vi "parse simple scan cluster.vi"(9 "variable":string, 10 "device":string, 11 "Scan setup":T1={"Scan Start"=1.0, "Scan End"=10.0, "Scan Step Size"=1.0, "# Shots Each Step"=10, "single direction?"=TRUE} {"Scan Start" format="%#.9p"; "Scan End" format="%#.9p"; "Scan Step Size" format="%#.9p"}) -> (1 "# shots":i32, 2 "bin group":i32[](array[numeric]), 3 "State(s) out":string)   [LabVIEW 2020]
uses:
  scan parameters.ctl
  <userlib>/_OpenG.lib/array/array.llb/Remove Duplicates from 1D Array (DBL)__ogtk.vi
panel:
  out "# shots 2":dbl
  out "vals to scan":dbl[](array[numeric])
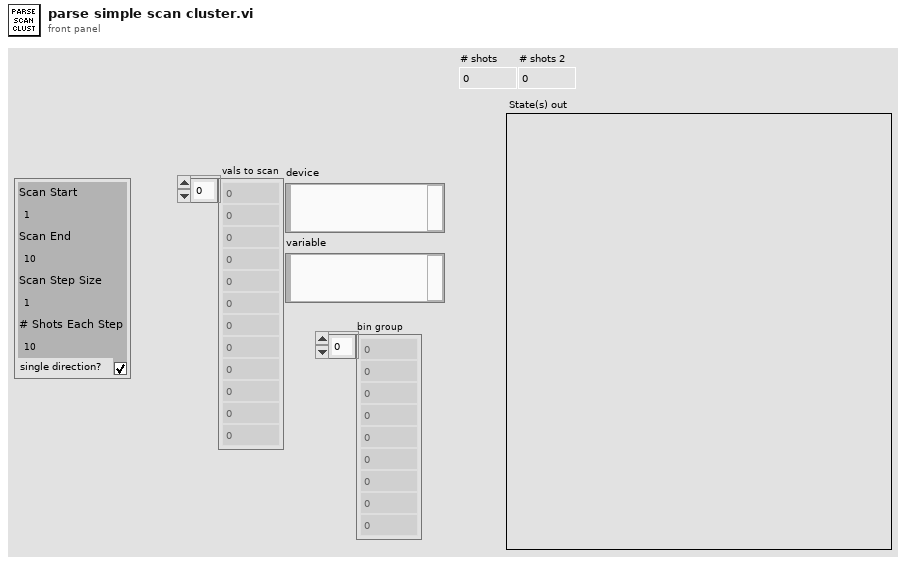
[diagram p1: front panel]
types:
  T1 = typedef "scan parameters.ctl" = cluster{"Scan Start":dbl, "Scan End":dbl, "Scan Step Size":dbl, "# Shots Each Step":u32, "single direction?":bool}
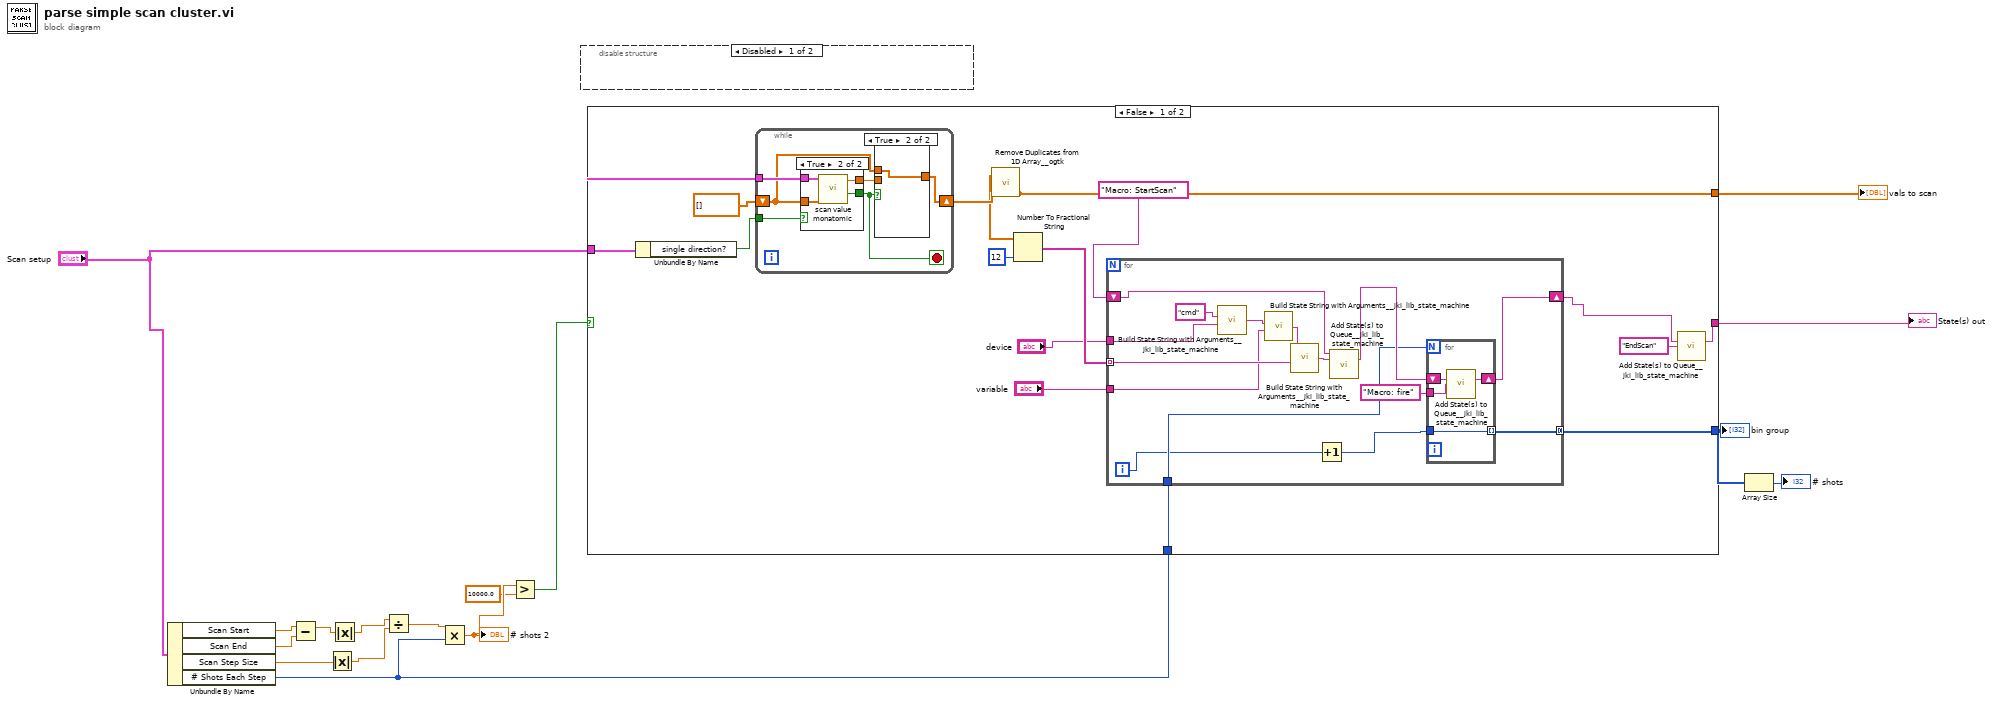
[diagram p0: block diagram]
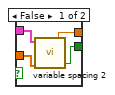
[diagram p2: hidden frame]
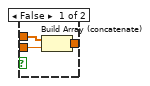
[diagram p3: hidden frame]
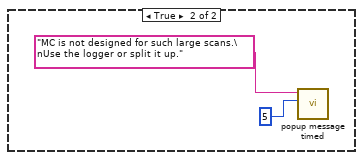
[diagram p4: hidden frame]
diagram:
  n1 = Unbundle By Name("Scan setup") -> ("Scan Start"=w12:dbl, "Scan End"=w11:dbl, "Scan Step Size"=w10:dbl, "# Shots Each Step"=w5:u32)
  n2 = Subtract(x=w12, y=w11) -> (x-y=w9:dbl)
  n3 = Absolute Value(x=w10) -> (abs(x)=w7:dbl)
  n4 = Absolute Value(x=w9) -> (abs(x)=w8:dbl)
  n5 = Divide(x=w8, y=w7) -> (x/y=w6:dbl)
  n6 = Multiply(x=w6, y=w5) -> (x*y=w4:dbl)
  "# shots 2" <- w4
  n7 = Greater?(x=w4, y=10000.0) -> (0:w2:bool)
  n8 = disable-structure shown="Disabled" {
    frame Disabled {
    }
    frame Enabled {
    }
  }
  n9 = case shown="False" w2 {
    tunnel: "Scan setup" -> [w31 _]
    tunnel: [w30 _] -> w15
    tunnel: [w24 _] -> w14
    tunnel: w5 -> [w20 _]
    tunnel: [w17 _] -> w1
    frame False {
      n10 = Unbundle By Name(w31) -> ("single direction?"=w25:bool)
      n11 = while {
        tunnel: w31 -> [w37]
        shift-right: [w34] -> w30
        shift-left: dbl[] [] ("parameter vals scanned") -> [w36]
        tunnel: w25 -> [w32]
        stop <- w33 stop-if-true
        n12 = case shown="True" w32 {
          tunnel: w37 -> [w41 w45]
          tunnel: w36 -> [w40 w44]
          tunnel: [w39 w43] -> w35
          tunnel: [w38 w42] -> w33
          frame False {
            n13 = call "variable spacing 2.vi"("shot times"=w40, "Scan parameters"=w41) -> ("quit"=w38:bool, "time aimed"=w39:dbl)  [unwired: 2 in, 1 out]
          }
          frame True {
            n14 = call "scan value monatomic.vi"("parameter vals scanned"=w44, "Scan parameters"=w45) -> ("scan complete"=w42:bool, "Next Value"=w43:dbl)  [unwired: 7 in, 1 out]
          }
        }
        n15 = case shown="True" w33 {
          tunnel: w36 -> [w48 w49]
          tunnel: w35 -> [w47 _]
          tunnel: [w46 w49] -> w34
          frame False {
            n16 = Build Array (concatenate)(w48, w47) -> (w46:dbl[])
          }
          frame True {
          }
        }
      }
      n17 = call-poly <userlib>:"Remove Duplicates from 1D Array__ogtk.vi"("Input Array"=w30) -> ("Output Array"=w29:dbl[])  [unwired: 1 out]
      n18 = Number To Fractional String(number=w29, precision (6)=i16 12) -> (F-format string=w28:string[])  [unwired: 2 in]
      n19 = for {
        tunnel: w20 -> [w55]
        tunnel: w28 -> [w58] mode=indexing
        shift-right: [w56] -> w18
        shift-left: "Macro: StartScan" ("State(s) in") -> [w57]
        tunnel: [w53] -> w24 mode=concatenating
        tunnel: "device" -> [w51]
        tunnel: "variable" -> [w50]
        i -> [w52]
        n20 = call <vilib>:"Build State String with Arguments__jki_lib_state_machine.vi"("Arguments (\"\")"=w51, "State"="cmd") -> ("State with Arguments"=w60:string)  [unwired: 4 in]
        n21 = call <vilib>:"Build State String with Arguments__jki_lib_state_machine.vi"("Arguments (\"\")"=w50, "State"=w60) -> ("State with Arguments"=w61:string)  [unwired: 4 in]
        n22 = call <vilib>:"Build State String with Arguments__jki_lib_state_machine.vi"("Arguments (\"\")"=w58, "State"=w61) -> ("State with Arguments"=w62:string)  [unwired: 4 in]
        n23 = Increment(x=w52) -> (x+1=w54:i32)
        n24 = call <vilib>:"Add State(s) to Queue__jki_lib_state_machine.vi"("State(s) in Front (\"\")"=w57, "State(s) in (\"\")"=w62) -> ("States Out"=w63:string)  [unwired: 13 in]
        n25 = for {
          N: w55 -> [_]
          shift-right: [w66] -> w56
          shift-left: w63 -> [w67]
          tunnel: "Macro: fire" ("Scan/Command") -> [w68]
          tunnel: w54 -> [w65]
          tunnel: [w65] -> w53 mode=indexing
          n26 = call <vilib>:"Add State(s) to Queue__jki_lib_state_machine.vi"("State(s) in (\"\")"=w67, "State(s) at Back (\"\")"=w68) -> ("States Out"=w66:string)  [unwired: 13 in]
        }
      }
      n27 = call <vilib>:"Add State(s) to Queue__jki_lib_state_machine.vi"("State(s) in (\"\")"=w18, "State(s) at Back (\"\")"="EndScan" ("State(s) at Back (\"\")")) -> ("States Out"=w17:string)  [unwired: 13 in]
    }
    frame True {
      n28 = call "popup message timed.vi"("seconds to wait"=u32 5, "Message:"="MC is not designed for such large scans.\nUse the logger or split it up.") -> ()  [unwired: 10 in]
    }
  }
  "vals to scan" <- w15
  "State(s) out" <- w1
  "bin group" <- w14
  n29 = Array Size(array=w14) -> (size(s)=→"# shots":i32)
